vi "OC2 Setup Setpoint.vi"(0 "VISA resource name":refnum<visa-resource-name>="ASRL1::INSTR", 1 "Setup setpoint values in":T1={"Setpoint"=0, "pot range"=100.0, "value"=25.0, "pot offset"=0.0, "X coeff deg/V"=100.0, "Rate deg/V"=25.0, "C coeff deg"=0.0} {"C coeff deg" format="%.2f"; "Rate deg/V" format="%.3f"; "X coeff deg/V" format="%.2f"; "pot offset" format="%.2f"; "value" format="%.3f"; "pot range" format="%.2f"; "Setpoint" items=["Pot", "Value"]}, 2 "error in (no error)":errorcluster, 4 "enable":bool) -> (3 "dup VISA resource name":refnum<visa-resource-name>, 5 "Setup setpoint values out":T1={"Setpoint"=0, "pot range"=100.0, "value"=25.0, "pot offset"=0.0, "X coeff deg/V"=100.0, "Rate deg/V"=25.0, "C coeff deg"=0.0} {"C coeff deg" format="%.2f"; "Rate deg/V" format="%.3f"; "X coeff deg/V" format="%.2f"; "pot offset" format="%.2f"; "value" format="%.3f"; "pot range" format="%.2f"; "Setpoint" items=["Pot", "Value"]}, 6 "error out":errorcluster)   [LabVIEW 2009]
doc: "TCM Setup Setpoint.vi\n\nVI that sets the setpoint information, accepts a cluster that contains the following variables:\nSetpoint control - Pot (on board TCM), value - user determined setpoint defined by value\nvalue - the value for the setpoint if valuye on setpointcontrol is set to value\npot range - the rsnge that the Pot on the TCM\npot offset - the offset of the pot\n\nCOPYRIGHT ELECTRON DYNAMICS LTD"
panel:
  out "write data":string
  # "Set setpoint variables"
  # "V1.02"
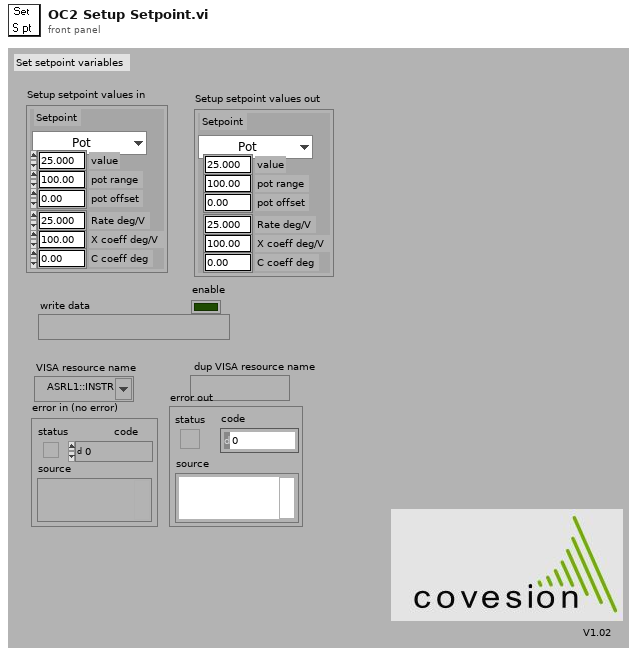
[diagram p1: front panel]
types:
  T1 = cluster{"Setpoint":u16, "pot range":dbl, "value":dbl, "pot offset":dbl, "X coeff deg/V":dbl, "Rate deg/V":dbl, "C coeff deg":dbl}
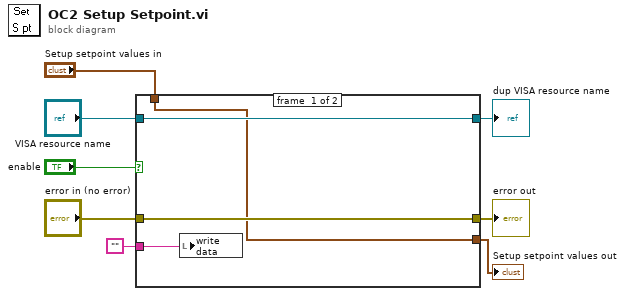
[diagram p0: block diagram]
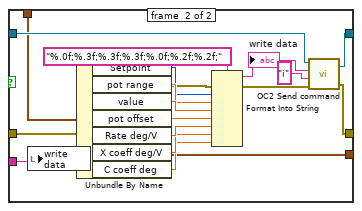
[diagram p2: hidden frame]
diagram:
  n1 = case shown="True" "enable" {
    tunnel: "VISA resource name" -> [w12 w27]
    tunnel: "error in (no error)" -> [w11 w14]
    tunnel: [w11 w26] -> w6
    tunnel: [w12 w25] -> w5
    tunnel: "" -> [w10 w24]
    tunnel: "Setup setpoint values in" -> [w9 w13]
    tunnel: [w9 w13] -> w2
    frame #0 {
      n2 = local write "write data"(w10) -> ()
    }
    frame #1 {
      n3 = local write "write data"(w24) -> ()
      n4 = Unbundle By Name(w13) -> ("Setpoint"=w18:u16, "pot range"=w19:dbl, "value"=w20:dbl, "pot offset"=w21:dbl, "Rate deg/V"=w17:dbl, "X coeff deg/V"=w16:dbl, "C coeff deg"=w15:dbl)
      n5 = Format Into String(format string="%.0f;%.3f;%.3f;%.3f;%.0f;%.2f;%.2f;", error in=w14, w18, w19, w20, w21, w17, w16, w15) -> (resulting string=w28:string, error out=w23:errorcluster)  [unwired: 1 in]
      "write data" <- w28
      n6 = call "OC2 Send command.vi"("VISA resource name"=w27, "Command data"=w28, "Command"="i", "error in (no error)"=w23) -> ("dup VISA resource name"=w25:refnum<visa-resource-name>, "error out"=w26:errorcluster)  [unwired: 1 in]
    }
  }
  "dup VISA resource name" <- w5
  "error out" <- w6
  "Setup setpoint values out" <- w2
